vi "Main.vi"(11 "Module Admin":refnum<class "Delacor_lib_QMH_Module Admin.lvclass">) -> ()   [LabVIEW 2024, in "ListViewer.lvlib"]
doc: "This template is based off of the Queued Message Handler design pattern and the Queued Message Handler project template that ships with LabVIEW.\n\nThe main difference is that the queue is private to this module and communication between modules is performed via Broadcast and Request events.\n\nRequest events are wrapped in public API methods and are handled in the Event Handling Loop (EHL) of this VI. Any module can register for Broadcast events sent by this module. The EHL generates messages based on user interface actions.\n\nThe Message Handling Loop (MHL) processes messages generated by the EHL, or by other messages. The messages are string values, so new messages can be added easily to the Message Cases case structure in the MHL. Each message cluster can also provide an optional value for Message Data, which is a variant that can be converted to whatever message-specific data is required.\n_____\nBased on DQMH Project Template 7.0.1.1316."
uses:
  ListViewer.lvlib
  <vilib>/Delacor/Delacor QMH/Libraries/Module Admin_class/Delacor_lib_QMH_Module Admin.lvclass
  Module Data--cluster.ctl
  Config.ctl
  <vilib>/Delacor/Delacor QMH/Libraries/Message Queue_class/Delacor_lib_QMH_Message Queue.lvclass/Delacor_lib_QMH_Message Queue.ctl
  Stop Argument--cluster.ctl
  <vilib>/Delacor/Delacor QMH/Libraries/Module Admin_class/Delacor_lib_QMH_Module Admin.lvclass/Delacor_lib_QMH_Module Admin.ctl
  Get UI Reference Argument--cluster.ctl
  Get UI Reference (Reply Payload)--cluster.ctl
  Inserted Into Subpanel Argument--cluster.ctl
  Set Config (String) Argument--cluster.ctl
  Set Config Argument--cluster.ctl
  Get config Argument--cluster.ctl
  Get config (Reply Payload)--cluster.ctl
  Get Config (String) Argument--cluster.ctl
  Get Config (String) (Reply Payload)--cluster.ctl
  <vilib>/Delacor/Delacor QMH/Libraries/Message Queue_class/Delacor_lib_QMH_Enqueue Message (Single).vi
  <vilib>/Delacor/Delacor QMH/Libraries/Module Admin_class/Delacor_lib_QMH_Get External Launch.vi
  <vilib>/Delacor/Delacor QMH/Libraries/Message Queue_class/Delacor_lib_QMH_Message Queue.lvclass
  <userlib>/_OpenG.lib/appcontrol/appcontrol.llb/openg_application_control.lvlib
panel:
  out "Title":string
  out "error out":errorcluster
  out "Status":string
  in  "Simulate MHL Error":bool
  in  "Simulate EHL Error":bool
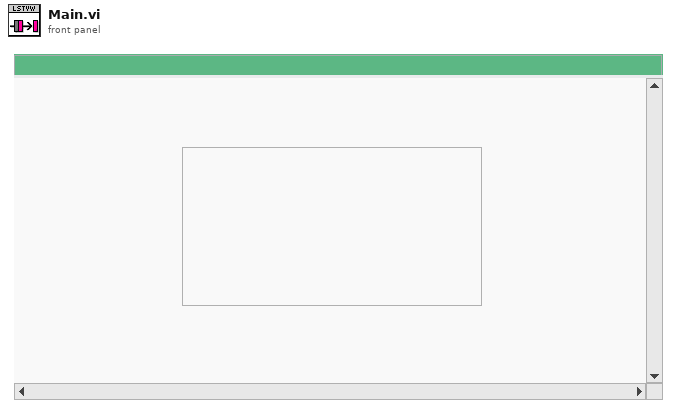
[diagram p1: front panel]
types:
  T1 = typedef "ListViewer.lvlib/Request Events--cluster.ctl" = cluster{"Stop Module":refnum<user-event>, "Show Panel":refnum<user-event>, "Hide Panel":refnum<user-event>, "Get Module Execution Status":refnum<user-event>, "Show Diagram":refnum<user-event>, "Get UI Reference":refnum<user-event>, "Inserted Into Subpanel":refnum<user-event>, "Set Config (String)":refnum<user-event>, "Set Config":refnum<user-event>, "Get config":refnum<user-event>, "Get Config (String)":refnum<user-event>}
  T2 = typedef "ListViewer.lvlib/Module Data--cluster.ctl" = cluster{"Status":string, "Config":T3}
  T3 = typedef "ListViewer.lvlib/Config.ctl" = cluster{"<ReplaceMe>":bool}
  T4 = enum32{"invalid lock state", "Not Locked", "Locked (No Password)", "Password-protected"}
  T5 = typedef "ListViewer.lvlib/Stop Argument--cluster.ctl" = cluster{"Origin":string, "Exit via Stop Module Req?":bool, "Wait for Module to stop?":bool}
  T6 = typedef "ListViewer.lvlib/Get UI Reference Argument--cluster.ctl" = cluster{"Wait Notifier":refnum<notifier>, "wait for reply":bool}
  T7 = typedef "ListViewer.lvlib/Inserted Into Subpanel Argument--cluster.ctl" = cluster{"Boolean":bool}
  T8 = typedef "ListViewer.lvlib/Set Config (String) Argument--cluster.ctl" = cluster{"XML-String":string}
  T9 = typedef "ListViewer.lvlib/Set Config Argument--cluster.ctl" = cluster{"Config":T3}
  T10 = typedef "ListViewer.lvlib/Get config Argument--cluster.ctl" = cluster{"Wait Notifier":refnum<notifier>, "wait for reply":bool}
  T11 = typedef "ListViewer.lvlib/Get Config (String) Argument--cluster.ctl" = cluster{"Wait Notifier":refnum<notifier>, "wait for reply":bool}
  T12 = enum32{"Invalid", "Standard", "Closed", "Hidden", "Minimized", "Maximized"}
  T13 = typedef "ListViewer.lvlib/Get UI Reference (Reply Payload)--cluster.ctl" = cluster{"UI VI Refnum":refnum<vi>, "error":errorcluster}
  T14 = typedef "ListViewer.lvlib/Get config (Reply Payload)--cluster.ctl" = cluster{"Config":T3, "error":errorcluster}
  T15 = typedef "ListViewer.lvlib/Get Config (String) (Reply Payload)--cluster.ctl" = cluster{"Config XML String":string, "error":errorcluster}
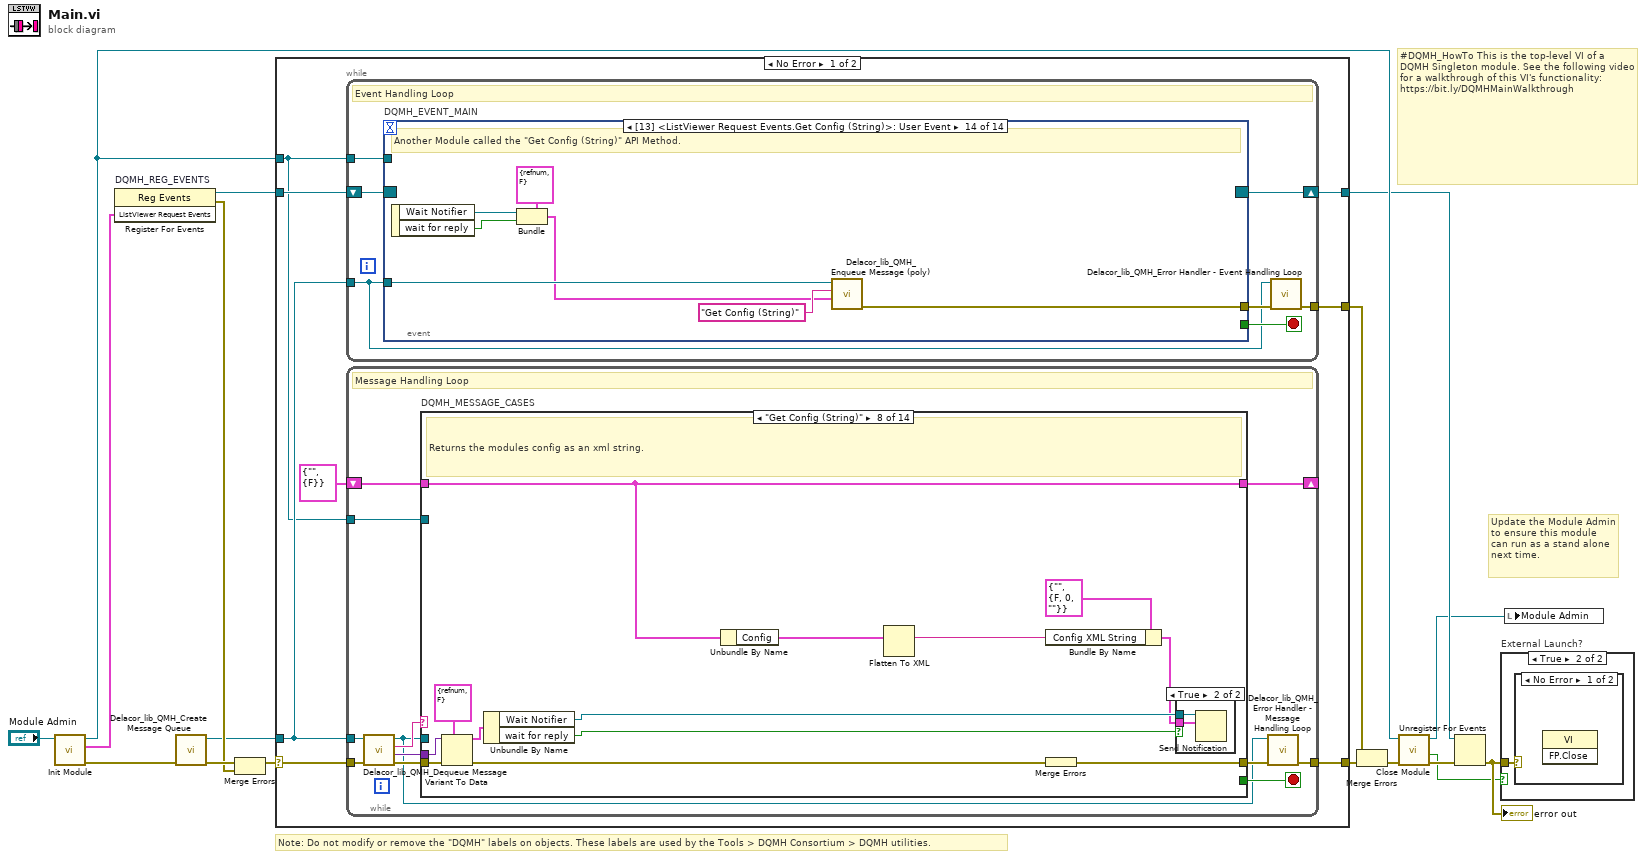
[diagram p0: block diagram]
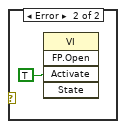
[diagram p3: hidden frame]
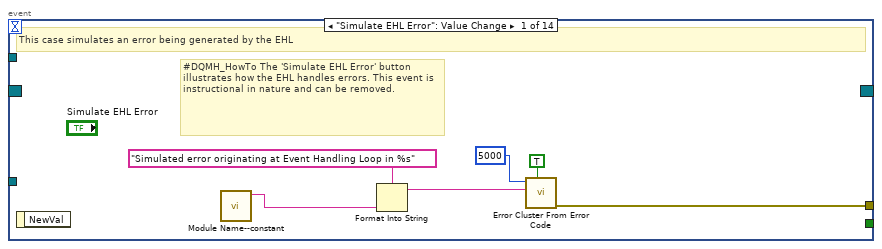
[diagram p4: hidden frame]
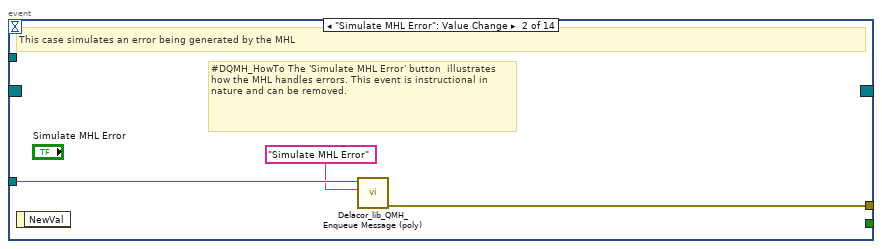
[diagram p5: hidden frame]
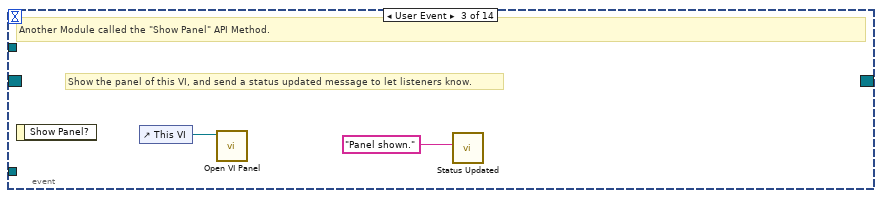
[diagram p6: hidden frame]
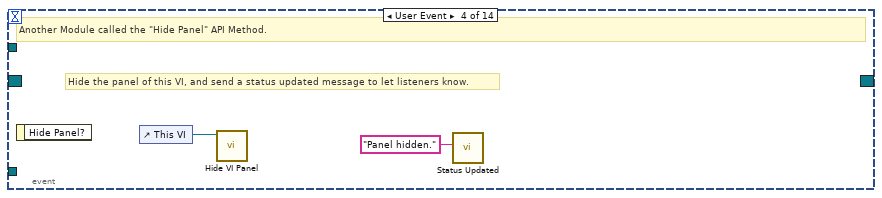
[diagram p7: hidden frame]
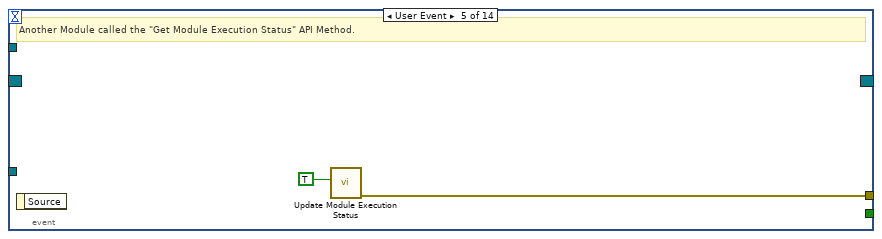
[diagram p8: hidden frame]
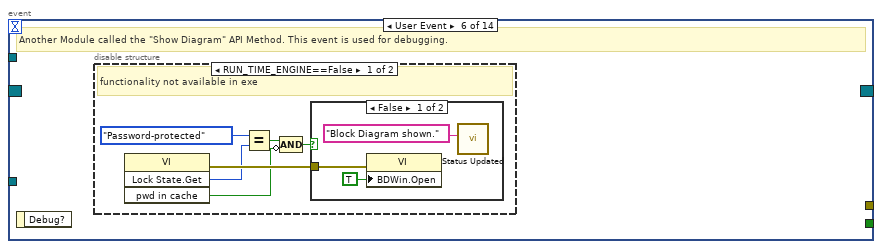
[diagram p9: hidden frame]
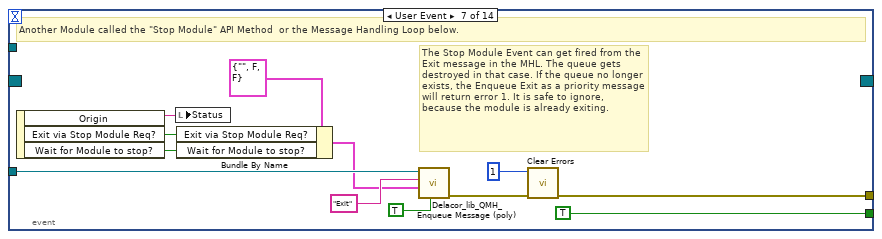
[diagram p12: hidden frame]
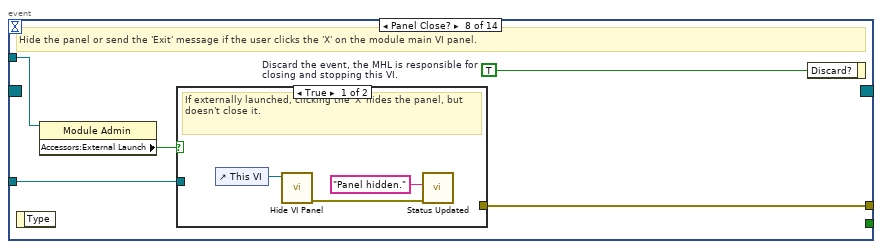
[diagram p13: hidden frame]
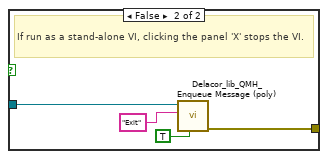
[diagram p14: hidden frame]
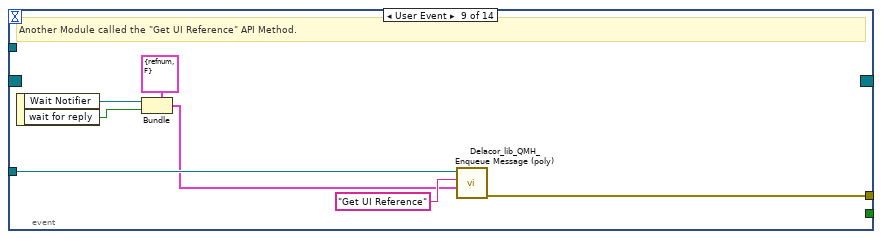
[diagram p15: hidden frame]
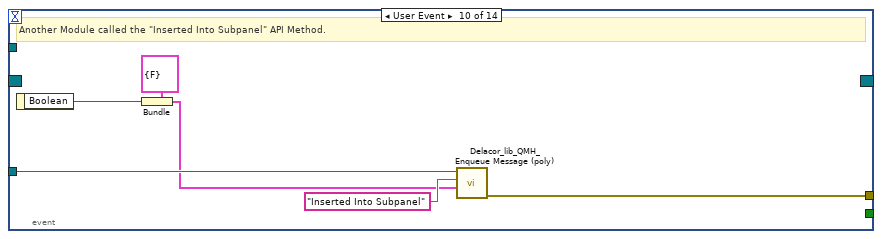
[diagram p16: hidden frame]
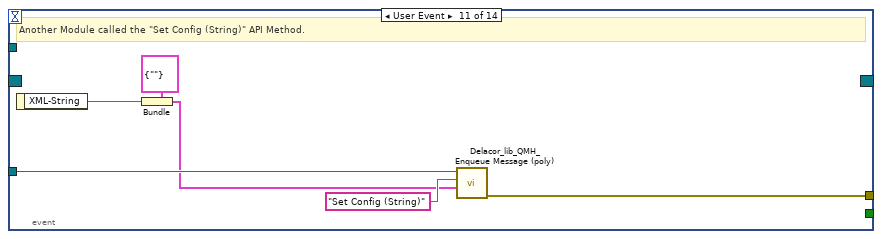
[diagram p17: hidden frame]
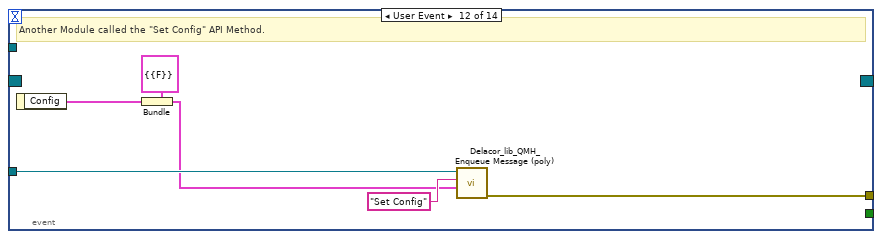
[diagram p18: hidden frame]
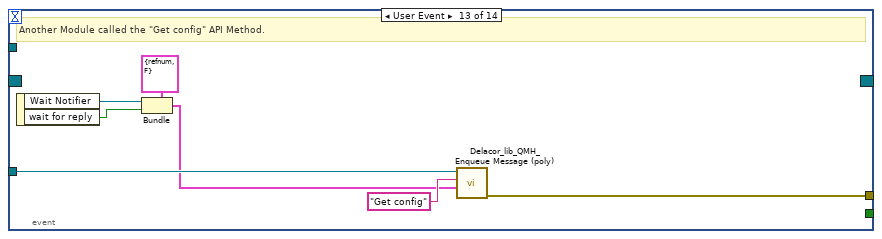
[diagram p19: hidden frame]
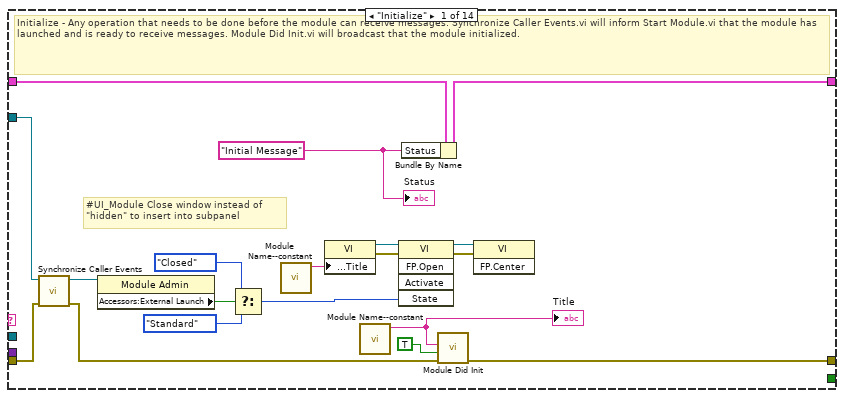
[diagram p20: hidden frame]
diagram:
  # "#DQMH_HowTo This is the top-level VI of a DQMH Singleton module. See the following video for a walkthrough of this VI's functionality: https://bit.ly/DQMHMainWalkthrough"
  # "Note: Do not modify or remove the \"DQMH\" labels on objects. These labels are used by the Tools > DQMH Consortium > DQMH utilities."
  # "Update the Module Admin to ensure this module can run as a stand alone next time."
  n1 = call "Init Module.vi"("Singleton Module Admin in"="Module Admin") -> ("error out"=w16:errorcluster, "ListViewer Request Events"=w5:T1, "Singleton Module Admin out"=w8:refnum<class "Delacor_lib_QMH_Module Admin.lvclass">)  [unwired: 8 in]
  n2 = register-events "DQMH_REG_EVENTS"(w5) -> (reference out=w6:refnum<event-registration>, error out=w9:errorcluster)  [unwired: 2 in]
  n3 = call <vilib>:"Delacor_lib_QMH_Create Message Queue.vi"("error in"=w16) -> ("error out"=w11:errorcluster, "Message Queue"=w4:refnum<class "Delacor_lib_QMH_Message Queue.lvclass">)  [unwired: 9 in]
  n4 = Merge Errors(w11, w9) -> (w10:errorcluster)
  n5 = case shown="No Error" w10 {
    selector: w10 -> [w23 w278]
    tunnel: [w25 w277] -> w17
    tunnel: [w22 w276] -> w7
    tunnel: w6 -> [w20 w276]
    tunnel: w4 -> [w19 w271]
    tunnel: [w24 _] -> w14
    tunnel: w8 -> [w18 w272]
    frame No Error {
      n6 = while {
        tunnel: w19 -> [w26]
        shift-right: [w29] -> w22
        shift-left: w20 -> [w30]
        tunnel: [w31] -> w24
        tunnel: w18 -> [w27]
        stop <- w28 stop-if-true
        # "Event Handling Loop"
        n7 = event "DQMH_EVENT_MAIN" shown="[13] <ListViewer Request Events.Get Config (String)>: User Event" {
          selector: w30 -> [_ _ _ _ _ _ _ _ _ _ _ _ _ _]
          dyn-events: [_ _ _ _ _ _ _ _ _ _ _ _ _ _] -> w29
          timeout: _ -> [_ _ _ _ _ _ _ _ _ _ _ _ _ _]
          tunnel: [_ _ _ _ _ _ TRUE ("Discard?") _ _ _ _ _ _ _] -> w28
          tunnel: w26 -> [_ w40 _ _ _ _ w64 w71 w87 w93 w99 w105 w112 w119]
          tunnel: [w38 w41 _ _ w47 _ w67 w73 w81 w88 w94 w100 w106 w113] -> w32
          tunnel: w27 -> [_ _ _ _ _ _ _ w70 _ _ _ _ _ _]
          event "Simulate EHL Error": Value Change {
            # "#DQMH_HowTo The 'Simulate EHL Error' button  illustrates how the EHL handles errors. This event is instructional in nature and can be removed."
            # "This case simulates an error being generated by the EHL"
            n8 = event-data() -> ()  [unwired: 1 in, 1 out]
            n9 = call "Module Name--constant.vi"() -> ("Module Name"=w35:string)  [unwired: 11 in]
            n10 = Format Into String(format string="Simulated error originating at Event Handling Loop in %s", w35) -> (resulting string=w36:string)  [unwired: 2 in, 1 out]
            n11 = call <vilib>:"Error Cluster From Error Code.vi"("show call chain? (False)"=TRUE, "error message (\"\")"=w36, "error code (0)"=5000) -> ("error out"=w38:errorcluster)  [unwired: 6 in]
          }
          event "Simulate MHL Error": Value Change {
            # "#DQMH_HowTo The 'Simulate MHL Error' button  illustrates how the MHL handles errors. This event is instructional in nature and can be removed."
            # "This case simulates an error being generated by the MHL"
            n12 = event-data() -> ()  [unwired: 1 in, 1 out]
            n13 = call-poly <vilib>:"Delacor_lib_QMH_Enqueue Message (poly).vi"("Message"="Simulate MHL Error", "Message Queue in"=w40) -> ("error out"=w41:errorcluster)  [unwired: 8 in, 1 out]
          }
          event User Event {
            # "Show the panel of this VI, and send a status updated message to let listeners know."
            # "Another Module called the \"Show Panel\" API Method."
            n14 = event-data() -> ()  [unwired: 1 in, 1 out]
            n15 = control-ref of="This VI"() -> (w43:refnum<vi>)
            n16 = call "Open VI Panel.vi"("VI"=w43) -> ()  [unwired: 10 in, 1 out]
            n17 = call "Status Updated.vi"("Status"="Panel shown." ("format string")) -> ()  [unwired: 10 in, 1 out]
          }
          event User Event {
            # "Hide the panel of this VI, and send a status updated message to let listeners know."
            # "Another Module called the \"Hide Panel\" API Method."
            n18 = event-data() -> ()  [unwired: 1 in, 1 out]
            n19 = control-ref of="This VI"() -> (w45:refnum<vi>)
            n20 = call "Hide VI Panel.vi"("VI"=w45) -> ()  [unwired: 10 in, 1 out]
            n21 = call "Status Updated.vi"("Status"="Panel hidden." ("format string")) -> ()  [unwired: 10 in, 1 out]
          }
          event User Event {
            # "Another Module called the \"Get Module Execution Status\" API Method."
            n22 = event-data() -> ()  [unwired: 1 in, 1 out]
            n23 = call "Update Module Execution Status.vi"("Running?"=TRUE) -> ("error out"=w47:errorcluster)  [unwired: 10 in]
          }
          event User Event {
            # "Another Module called the \"Show Diagram\" API Method. This event is used for debugging."
            n24 = event-data() -> ()  [unwired: 1 in, 1 out]
            n25 = disable-structure shown="RUN_TIME_ENGINE==False" {
              frame condition #0 (active) {
                # "functionality not available in exe"
                n26 = invoke on="Invoke Node" class="VI" method="Lock State.Get"() -> (error out=w53:errorcluster, "Get Lock State"=w52:T4, "pwd in cache"=w49:bool)  [unwired: 4 in, 1 out]
                n27 = Equal?(x=T4."Password-protected", y=w52) -> (x = y?=w50:bool)
                n28 = Compound Arithmetic op=AND(w50, invert w49) -> (w48:bool)
                n29 = case shown="False" w48 {
                  tunnel: w53 -> [w56 _]
                  frame False {
                    n30 = property on="Property Node" class="VI"(error in=w56, "BDWin.Open"=TRUE ("Block Diagram Window:Open")) -> ()  [unwired: 1 in, 2 out]
                    n31 = call "Status Updated.vi"("Status"="Block Diagram shown." ("format string")) -> ()  [unwired: 10 in, 1 out]
                  }
                  frame True {
                    # "Password-protected VI, and the password is not in the cache. Do not show the diagram."
                  }
                }
              }
              frame condition #1 {
              }
            }
          }
          event User Event {
            # "The Stop Module Event can get fired from the Exit message in the MHL. The queue gets destroyed in that case. If the queue no longer exists, the Enqueue Exit as a priority message will return error 1. It is safe to ignore, because the module is already exiting."
            # "Another Module called the \"Stop Module\" API Method  or the Message Handling Loop below."
            n32 = event-data() -> ("Origin"=w63:string, "Exit via Stop Module Req?"=w59:bool, "Wait for Module to stop?"=w58:bool)  [unwired: 1 in]
            n33 = local write "Status"(w63) -> ()
            n34 = Bundle By Name(cluster=T5 {"Origin"="", "Exit via Stop Module Req?"=FALSE, "Wait for Module to stop?"=FALSE} ("Stop Argument"), "Exit via Stop Module Req?"=w59, "Wait for Module to stop?"=w58) -> (w57:T5)
            n35 = call-poly <vilib>:"Delacor_lib_QMH_Enqueue Message (poly).vi"("Priority Message? (F)"=TRUE, "Message Data"=w57, "Message"="Exit", "Message Queue in"=w64) -> ("error out"=w68:errorcluster)  [unwired: 6 in, 1 out]
            n36 = call <vilib>:"Clear Errors.vi"("error in (no error)"=w68, "specific error code to clear (0: all)"=1) -> ("error out"=w67:errorcluster)  [unwired: 4 in, 1 out]
          }
          event Panel Close? {
            w72 = TRUE  # Discard the event, the MHL is responsible for closing and stopping this VI.
            # "Hide the panel or send the 'Exit' message if the user clicks the 'X' on the module main VI panel."
            n37 = event-data() -> ()  [unwired: 1 in, 1 out]
            n38 = property on="Property Node" class="Module Admin"(reference=w70) -> ("Accessors:External Launch"=w69:bool)  [unwired: 1 in, 2 out]
            n39 = case shown="True" w69 {
              tunnel: w71 -> [_ w79]
              tunnel: [_ w80] -> w73
              frame True {
                # "If externally launched, clicking the 'X' hides the panel, but doesn't close it."
                n40 = control-ref of="This VI"() -> (w76:refnum<vi>)
                n41 = call "Hide VI Panel.vi"("VI"=w76) -> ("error out"=w74:errorcluster)  [unwired: 10 in]
                n42 = call "Status Updated.vi"("error in"=w74, "Status"="Panel hidden." ("format string")) -> ()  [unwired: 9 in, 1 out]
              }
              frame False {
                # "If run as a stand-alone VI, clicking the panel 'X' stops the VI."
                n43 = call-poly <vilib>:"Delacor_lib_QMH_Enqueue Message (poly).vi"("Priority Message? (F)"=TRUE, "Message"="Exit", "Message Queue in"=w79) -> ("error out"=w80:errorcluster)  [unwired: 7 in, 1 out]
              }
            }
            n44 = event-data ("Event Filter Node")("Discard?"=w72) -> ()  [unwired: 1 in, 1 out]
          }
          event User Event {
            # "Another Module called the \"Get UI Reference\" API Method."
            n45 = event-data() -> ("Wait Notifier"=w83:refnum<notifier>, "wait for reply"=w82:bool)  [unwired: 1 in]
            n46 = Bundle(cluster=T6 {"Wait Notifier"=refnum, "wait for reply"=FALSE} ("Get UI Reference Argument"), "Wait Notifier"=w83, "wait for reply"=w82) -> (w84:T6)
            n47 = call-poly <vilib>:"Delacor_lib_QMH_Enqueue Message (poly).vi"("Message Data"=w84, "Message"="Get UI Reference", "Message Queue in"=w87) -> ("error out"=w81:errorcluster)  [unwired: 7 in, 1 out]
          }
          event User Event {
            # "Another Module called the \"Inserted Into Subpanel\" API Method."
            n48 = event-data() -> ("Boolean"=w89:bool)  [unwired: 1 in]
            n49 = Bundle(cluster=T7 {"Boolean"=FALSE} ("Inserted Into Subpanel Argument"), "Boolean"=w89) -> (w90:T7)
            n50 = call-poly <vilib>:"Delacor_lib_QMH_Enqueue Message (poly).vi"("Message Data"=w90, "Message"="Inserted Into Subpanel", "Message Queue in"=w93) -> ("error out"=w88:errorcluster)  [unwired: 7 in, 1 out]
          }
          event User Event {
            # "Another Module called the \"Set Config (String)\" API Method."
            n51 = event-data() -> ("XML-String"=w95:string)  [unwired: 1 in]
            n52 = Bundle(cluster=T8 {"XML-String"=""} ("Set Config (String) Argument"), "XML-String"=w95) -> (w96:T8)
            n53 = call-poly <vilib>:"Delacor_lib_QMH_Enqueue Message (poly).vi"("Message Data"=w96, "Message"="Set Config (String)", "Message Queue in"=w99) -> ("error out"=w94:errorcluster)  [unwired: 7 in, 1 out]
          }
          event User Event {
            # "Another Module called the \"Set Config\" API Method."
            n54 = event-data() -> ("Config"=w101:T3)  [unwired: 1 in]
            n55 = Bundle(cluster=T9 {"Config"={"<ReplaceMe>"=FALSE}} ("Set Config Argument"), "Config"=w101) -> (w102:T9)
            n56 = call-poly <vilib>:"Delacor_lib_QMH_Enqueue Message (poly).vi"("Message Data"=w102, "Message"="Set Config", "Message Queue in"=w105) -> ("error out"=w100:errorcluster)  [unwired: 7 in, 1 out]
          }
          event User Event {
            # "Another Module called the \"Get config\" API Method."
            n57 = event-data() -> ("Wait Notifier"=w108:refnum<notifier>, "wait for reply"=w107:bool)  [unwired: 1 in]
            n58 = Bundle(cluster=T10 {"Wait Notifier"=refnum, "wait for reply"=FALSE} ("Get config Argument"), "Wait Notifier"=w108, "wait for reply"=w107) -> (w109:T10)
            n59 = call-poly <vilib>:"Delacor_lib_QMH_Enqueue Message (poly).vi"("Message Data"=w109, "Message"="Get config", "Message Queue in"=w112) -> ("error out"=w106:errorcluster)  [unwired: 7 in, 1 out]
          }
          event User Event {
            # "Another Module called the \"Get Config (String)\" API Method."
            n60 = event-data() -> ("Wait Notifier"=w115:refnum<notifier>, "wait for reply"=w114:bool)  [unwired: 1 in]
            n61 = Bundle(cluster=T11 {"Wait Notifier"=refnum, "wait for reply"=FALSE} ("Get Config (String) Argument"), "Wait Notifier"=w115, "wait for reply"=w114) -> (w116:T11)
            n62 = call-poly <vilib>:"Delacor_lib_QMH_Enqueue Message (poly).vi"("Message Data"=w116, "Message"="Get Config (String)", "Message Queue in"=w119) -> ("error out"=w113:errorcluster)  [unwired: 7 in, 1 out]
          }
        }
        n63 = call-dynamic "Delacor_lib_QMH_Error Handler - Event Handling Loop.vi"("error in"=w32, "Message Queue in"=w26) -> ("dup error in"=w31:errorcluster)  [unwired: 8 in, 1 out]
      }
      n64 = while {
        tunnel: w19 -> [w120]
        shift-right: [w128] -> _
        shift-left: T2 {"Status"="", "Config"={"<ReplaceMe>"=FALSE}} ("Data Cluster") -> [w129]
        tunnel: w23 -> [w131]
        tunnel: [w123] -> w25
        tunnel: w18 -> [w124]
        stop <- w127 stop-if-true
        # "Message Handling Loop"
        n65 = call-dynamic "Delacor_lib_QMH_Dequeue Message.vi"("error in"=w131, "Message Queue in"=w120) -> ("error out"=w130:errorcluster, "Message Data"=w125:variant, "Message"=w126:string, "Message Queue out"=w121:refnum<class "Delacor_lib_QMH_Message Queue.lvclass">)  [unwired: 6 in]
        n66 = case "DQMH_MESSAGE_CASES" shown="\"Get Config (String)\"" w126 {
          selector: w126 -> [_ _ _ _ _ _ _ _ _ _ _ _ _ w266]
          tunnel: w121 -> [_ _ _ _ _ _ _ _ _ _ _ w232 w254 _]
          tunnel: w130 -> [w148 w152 w164 w167 w179 w185 w197 w212 w217 w219 w228 w239 w260 w269]
          tunnel: [w146 w152 w154 w167 w173 w183 w188 w203 w216 w219 w227 w235 w255 w270] -> w122
          tunnel: w129 -> [w137 w151 w163 w168 w178 w184 w187 w202 w215 w218 w225 w234 w253 w267]
          tunnel: [w136 w151 w163 w168 w170 w184 w187 w202 w215 w218 w225 w234 w253 w267] -> w128
          tunnel: [_ _ _ _ _ _ _ _ _ _ _ _ w252 _] -> w127
          tunnel: w125 -> [_ _ w161 _ w176 w182 w195 w210 _ _ _ w233 w251 _]
          tunnel: w124 -> [w138 _ _ _ _ _ _ _ _ _ _ w231 w246 _]
          frame "Initialize" {
            w133 = "Initial Message" ("Initial Message")
            # "#UI_Module Close window instead of\n\"hidden\" to insert into subpanel"
            # "Initialize - Any operation that needs to be done before the module can receive messages. Synchronize Caller Events.vi will inform Start Module.vi that the module has launched and is ready to receive messages. Module Did Init.vi will broadcast that the module initialized."
            n67 = call "Synchronize Caller Events.vi"("error in"=w148, "Singleton Module Admin in"=w138) -> ("error out"=w147:errorcluster, "Singleton Module Admin out"=w134:refnum<class "Delacor_lib_QMH_Module Admin.lvclass">)  [unwired: 8 in]
            n68 = property on="Property Node" class="Module Admin"(reference=w134) -> ("Accessors:External Launch"=w142:bool)  [unwired: 1 in, 2 out]
            n69 = Select(t=T12."Closed" ("State"), s=w142, f=T12."Standard" ("State")) -> (s? t:f=w139:T12)
            n70 = call "Module Name--constant.vi"() -> ("Module Name"=w145:string)  [unwired: 11 in]
            n71 = property on="Property Node" class="VI"("Front Panel.Title"=w145) -> (reference out=w144:refnum<vi>, error out=w150:errorcluster)  [unwired: 2 in]
            n72 = call "Module Name--constant.vi"() -> ("Module Name"=w132:string)  [unwired: 11 in]
            "Title" <- w132
            n73 = invoke on="Invoke Node" class="VI" method="FP.Open"(reference=w144, error in=w150, "State"=w139) -> (reference out=w143:refnum<vi>, error out=w149:errorcluster)  [unwired: 2 in, 3 out]
            n74 = Bundle By Name(cluster=w137, "Status"=w133) -> (w136:T2)
            n75 = call "Module Did Init.vi"("error in"=w147, "Initialized?"=TRUE, "Origin"=w132) -> ("error out"=w146:errorcluster)  [unwired: 8 in]
            n76 = invoke on="Invoke Node" class="VI" method="FP.Center"(reference=w143, error in=w149) -> ()  [unwired: 1 in, 3 out]
            "Status" <- w133
          }
          frame "---Module Specific---" {
            # "Separator -- The following cases handle messages specific to this Module."
          }
          frame "Get UI Reference" {
            # "Returns the VI Reference of the UI of the Module, usually the main.vi. Use this to insert the Module into a sub-panel."
            n77 = Variant To Data(error in=w164, type=T6 {"Wait Notifier"=refnum, "wait for reply"=FALSE} ("Get UI Reference Argument"), Variant=w161) -> (data=w159:T6, error out=w162:errorcluster)
            n78 = Unbundle By Name(w159) -> ("Wait Notifier"=w158:refnum<notifier>, "wait for reply"=w157:bool)
            n79 = call <userlib>:"Current VIs Reference__ogtk.vi"() -> ("Current VI's reference"=w153:refnum<vi>)  [unwired: 5 in]
            n80 = Bundle By Name(cluster=T13 {"UI VI Refnum"=refnum, "error"={"status"=FALSE, "code"=0, "source"=""}} ("Get UI Reference (Reply Payload)"), "UI VI Refnum"=w153) -> (w156:T13)
            n81 = Merge Errors(w162) -> (w154:errorcluster)
            n82 = case "DQMH_FIRE_NOTIFIER" shown="True" w157 {
              tunnel: w158 -> [_ w166]
              tunnel: w156 -> [_ w165]
              frame False {
              }
              frame True {
                n83 = Send Notification(notification=w165, notifier=w166) -> ()  [unwired: 1 in, 2 out]
              }
            }
          }
          frame "Inserted Into Subpanel" {
            # "#UI_Module Update UI when inserted into a subpanel"
            # "This Request is called when the UI VI is inserted into a subpanel."
          }
          frame "Set Config (String)" {
            # "Sets the config data by String of the flattened config.ctl cluster."
            n84 = Variant To Data(error in=w179, type=T8 {"XML-String"=""} ("Set Config (String) Argument"), Variant=w176) -> (data=w174:T8, error out=w177:errorcluster)
            n85 = Unbundle By Name(w174) -> ("XML-String"=w172:string)
            n86 = Unflatten From XML(xml string=w172, type=T3 {"<ReplaceMe>"=FALSE} ("Config"), error in (no error)=w177) -> (value=w169:T3, error out=w173:errorcluster)
            n87 = Bundle By Name(cluster=w178, "Config"=w169) -> (w170:T2)
          }
          frame "Set Config" {
            # "#CodeNeeded\n1. Configure this Message Case for handling the \"Set Config\" message.\n2. Delete or edit this label when done."
            # "Sets the config data for the module."
            n88 = Variant To Data(error in=w185, type=T9 {"Config"={"<ReplaceMe>"=FALSE}} ("Set Config Argument"), Variant=w182) -> (data=w180:T9, error out=w183:errorcluster)
            n89 = Unbundle By Name(w180) -> ()  [unwired: 1 out]
          }
          frame "Get config" {
            # "Returns the modules Config."
            n90 = Variant To Data(error in=w197, type=T10 {"Wait Notifier"=refnum, "wait for reply"=FALSE} ("Get config Argument"), Variant=w195) -> (data=w193:T10, error out=w196:errorcluster)
            n91 = Unbundle By Name(w193) -> ("Wait Notifier"=w192:refnum<notifier>, "wait for reply"=w191:bool)
            n92 = Unbundle By Name(w187) -> ("Config"=w186:T3)
            n93 = Bundle By Name(cluster=T14 {"Config"={"<ReplaceMe>"=FALSE}, "error"={"status"=FALSE, "code"=0, "source"=""}} ("Get config (Reply Payload)"), "Config"=w186) -> (w190:T14)
            n94 = Merge Errors(w196) -> (w188:errorcluster)
            n95 = case "DQMH_FIRE_NOTIFIER" shown="True" w191 {
              tunnel: w192 -> [_ w199]
              tunnel: w190 -> [_ w198]
              frame False {
              }
              frame True {
                n96 = Send Notification(notification=w198, notifier=w199) -> ()  [unwired: 1 in, 2 out]
              }
            }
          }
          frame "Get Config (String)" {
            # "Returns the modules config as an xml string."
            n97 = Variant To Data(error in=w212, type=T11 {"Wait Notifier"=refnum, "wait for reply"=FALSE} ("Get Config (String) Argument"), Variant=w210) -> (data=w208:T11, error out=w211:errorcluster)
            n98 = Unbundle By Name(w208) -> ("Wait Notifier"=w207:refnum<notifier>, "wait for reply"=w206:bool)
            n99 = Unbundle By Name(w202) -> ("Config"=w201:T3)
            n100 = Flatten To XML(6:w201) -> (2:w200:string)
            n101 = Bundle By Name(cluster=T15 {"Config XML String"="", "error"={"status"=FALSE, "code"=0, "source"=""}} ("Get Config (String) (Reply Payload)"), "Config XML String"=w200) -> (w205:T15)
            n102 = Merge Errors(w211) -> (w203:errorcluster)
            n103 = case "DQMH_FIRE_NOTIFIER" shown="True" w206 {
              tunnel: w207 -> [_ w214]
              tunnel: w205 -> [_ w213]
              frame False {
              }
              frame True {
                n104 = Send Notification(notification=w213, notifier=w214) -> ()  [unwired: 1 in, 2 out]
              }
            }
          }
          frame "---Copy This Frame---" {
            # "Duplicate this frame when creating new messages.  Change this comment in the duplicated frame to describe this message."
            n105 = Merge Errors(w217) -> (w216:errorcluster)
          }
          frame "---Exit and Error Handling---" {
            # "Separator - The following cases handle errors and exit messages."
          }
          frame "Simulate MHL Error" {
            # "#DQMH_HowTo The 'Simulate MHL Error' button  illustrates how the MHL handles errors. This event is instructional in nature and can be removed."
            # "Simulate an error occurring at the MHL"
            n106 = call "Module Name--constant.vi"() -> ("Module Name"=w221:string)  [unwired: 11 in]
            n107 = Format Into String(format string="Simulated error originating at Message Handling Loop in %s", w221) -> (resulting string=w222:string)  [unwired: 2 in, 1 out]
            n108 = call <vilib>:"Error Cluster From Error Code.vi"("show call chain? (False)"=TRUE, "error message (\"\")"=w222, "error code (0)"=5001) -> ("error out"=w226:errorcluster)  [unwired: 6 in]
            n109 = Merge Errors(w228, w226) -> (w227:errorcluster)
          }
          frame "Error" {
            # "Error - Check the error message data and respond accordingly. This message is sent by the \"Error Handler\" VIs at the end of each loop in this application."
            n110 = property on="Property Node" class="Module Admin"(reference=w231) -> ("Accessors:External Launch"=w230:bool)  [unwired: 1 in, 2 out]
            n111 = Variant To Data(error in=w239, type=errorcluster {"status"=FALSE, "code"=0, "source"=""} ("error constant"), Variant=w233) -> (data=w229:errorcluster, error out=w237:errorcluster)
            n112 = local write "error out"(w229) -> ()
            n113 = call "Error Reported.vi"("Error"=w229) -> ()  [unwired: 10 in, 1 out]
            n114 = case shown="False" w230 {
              tunnel: [w244 _] -> w236
              tunnel: w232 -> [w242 _]
              tunnel: w229 -> [w243 _]
              frame False {
                n115 = disable-structure shown="Default" {
                  disable-tunnel: w243 -> [w245 _]
                  frame condition #0 (active) {
                    # "If the module is running standalone, then pop up an error dialog and call the \"Exit\" message."
                    n116 = call <vilib>:"Simple Error Handler.vi"("error in (no error)"=w245) -> ()  [unwired: 4 in, 5 out]
                  }
                  frame condition #1 {
                    # "To prevent the Simple Error Handler VI from being loaded (e.g. when deploying to a Real-Time target), add the Conditional Disable Symbol \"DQMH_Disable_SEH\" to your project and set it to TRUE."
                  }
                }
                n117 = call-poly <vilib>:"Delacor_lib_QMH_Enqueue Message (poly).vi"("Priority Message? (F)"=TRUE, "Message"="Exit", "Message Queue in"=w242) -> ("error out"=w244:errorcluster)  [unwired: 7 in, 1 out]
              }
              frame True {
                # "If the module was launched externally, calling the Error Reported broadcast VI is the only action performed by the \"Error\" message. The module's caller can then process the error appropriately."
              }
            }
            n118 = Merge Errors(w237, w236) -> (w235:errorcluster)
          }
          frame "Exit" {
            w250 = 91  # 91: not all Exit messages will have an argument
            w252 = TRUE  # Stop the VI
            # "Release the message queue reference"
            # "Exit - Exit the application."
            n119 = Variant To Data(error in=w260, type=T5 {"Origin"="", "Exit via Stop Module Req?"=FALSE, "Wait for Module to stop?"=FALSE} ("Stop Argument"), Variant=w251) -> (data=w248:T5, error out=w257:errorcluster)
            n120 = call <vilib>:"Clear Errors.vi"("error in (no error)"=w257, "specific error code to clear (0: all)"=w250) -> ("error out"=w259:errorcluster)  [unwired: 4 in, 1 out]
            n121 = control-ref of="This VI"() -> (w247:refnum<vi>)
            n122 = call-dynamic "Delacor_lib_QMH_Release Message Queue.vi"("error in"=w259, "Message Queue"=w254) -> ("error out"=w258:errorcluster)  [unwired: 9 in]
            n123 = call "Handle Exit.vi"("Stop Argument"=w248, "Admin in"=w246, "VI reference"=w247) -> ("error out"=w256:errorcluster)  [unwired: 7 in, 1 out]
            n124 = Merge Errors(w258, w256) -> (w255:errorcluster)
            n125 = call "Error Reported.vi"("Error"=w255) -> ()  [unwired: 10 in, 1 out]
          }
          frame Default {
            # "'Default' case only runs if there is a message that isn't defined in any of the other cases.  Output a programming error."
            n126 = call "Module Name--constant.vi"() -> ("Module Name"=w265:string)  [unwired: 11 in]
            n127 = Format Into String(format string="The invalid message string \"%s\" was received in the Message Handling Loop for module \"%s\".", w266, w265) -> (resulting string=w261:string)  [unwired: 2 in, 1 out]
            n128 = call <vilib>:"Error Cluster From Error Code.vi"("show call chain? (False)"=TRUE, "error message (\"\")"=w261, "error code (0)"=1) -> ("error out"=w268:errorcluster)  [unwired: 6 in]
            n129 = Merge Errors(w269, w268) -> (w270:errorcluster)
          }
        }
        n130 = call-dynamic "Delacor_lib_QMH_Error Handler - Message Handling Loop.vi"("error in"=w122, "Message Queue in"=w121) -> ("dup error in"=w123:errorcluster)  [unwired: 8 in, 1 out]
      }
    }
    frame Error {
      # "Synchronize Caller Events.vi will inform Start Module.vi that the module has launched and will let the code calling Start Module.vi register for broadcasts and would permit the caller receive the broadcast that an error occurred at launch time."
      n131 = call-dynamic "Delacor_lib_QMH_Release Message Queue.vi"("error in"=w278, "Message Queue"=w271) -> ("error out"=w277:errorcluster)  [unwired: 9 in]
      n132 = call "Synchronize Caller Events.vi"("Singleton Module Admin in"=w272) -> ("error out"=w279:errorcluster)  [unwired: 9 in, 1 out]
      n133 = call "Module Name--constant.vi"() -> ("Module Name"=w275:string)  [unwired: 11 in]
      n134 = Format Into String(format string="An error occurred during initialization. %s is no longer running.", w275) -> (resulting string=w273:string)  [unwired: 2 in, 1 out]
      n135 = Merge Errors(w277, w279) -> (w280:errorcluster)
      n136 = call "Error Reported.vi"("Additional Information"=w273, "Error"=w280) -> ()  [unwired: 9 in, 1 out]
    }
  }
  n137 = Merge Errors(w14, w17) -> (w13:errorcluster)
  n138 = call "Close Module.vi"("error in"=w13, "Module Admin in"=w8) -> ("error out"=w15:errorcluster, "External Launch"=w1:bool, "Module Admin out"=w2:refnum<class "Delacor_lib_QMH_Module Admin.lvclass">)  [unwired: 7 in]
  n139 = Unregister For Events(event registration refnum=w7, error in=w15) -> (error out=w12:errorcluster)
  "error out" <- w12
  n140 = case "External Launch?" shown="True" w1 {
    tunnel: w12 -> [_ w281]
    frame False {
    }
    frame True {
      n141 = case shown="No Error" w281 {
        frame No Error {
          n142 = invoke on="Invoke Node" class="VI" method="FP.Close"() -> ()  [unwired: 3 in, 3 out]
        }
        frame Error {
          n143 = invoke on="Invoke Node" class="VI" method="FP.Open"("Activate"=TRUE ("Activate?")) -> ()  [unwired: 4 in, 5 out]
        }
      }
    }
  }
  n144 = local write "Module Admin"(w2) -> ()
